vi "TestSpeedCache.vi"() -> ()   [LabVIEW 2017]
uses:
  <vilib>/addons/InsightCM/Utilities/Analysis/Shared/controls/SpeedCache.ctl
  <vilib>/addons/InsightCM/Utilities/Analysis/Shared/controls/SpeedCacheOps.ctl
  <vilib>/addons/InsightCM/Utilities/Analysis/Shared/AnalysisHelper.lvlib
panel:
  out "speed (RPM) 11":dbl
  out "pulse cache 11":T1
  in  "pulse position data 11":dbl[](array[numeric])
  out "speed (RPM) 10":dbl
  out "speed (RPM) 9":dbl
  out "pulse cache 10":T1
  out "pulse cache 9":T1
  in  "pulse position data 10":dbl[](array[numeric])
  in  "pulse position data 9":dbl[](array[numeric])
  out "pulse cache":T1
  out "Speed (RPM) 8":dbl
  out "Pulse Cache Type 8":T1
  in  "pulse position data 8":dbl[](array[numeric])
  in  "pulse position data 7":dbl[](array[numeric])
  out "Speed (RPM) 7":dbl
  out "Pulse Cache Type 7":T1
  out "Pulse Cache Type 6":T1
  out "Pulse Cache Type 5":T1
  out "Pulse Cache Type 4":T1
  out "Pulse Cache Type 3":T1
  out "Pulse Cache Type 2":T1
  out "Pulse Cache Type":T1
  out "Speed (RPM) 6":dbl
  out "Speed (RPM) 5":dbl
  out "Speed (RPM) 4":dbl
  in  "pulse position data 6":dbl[](array[numeric])
  in  "pulse position data 5":dbl[](array[numeric])
  in  "pulse position data 4":dbl[](array[numeric])
  out "Speed (RPM) 3":dbl
  out "Speed (RPM) 2":dbl
  out "Speed (RPM)":dbl
  in  "pulse position data 3":dbl[](array[numeric])
  in  "pulse position data 2":dbl[](array[numeric])
  in  "pulse position data":dbl[](array[numeric])
  # "120"
  # "40"
  # "30"
  # "40"
  # "24"
  # "20"
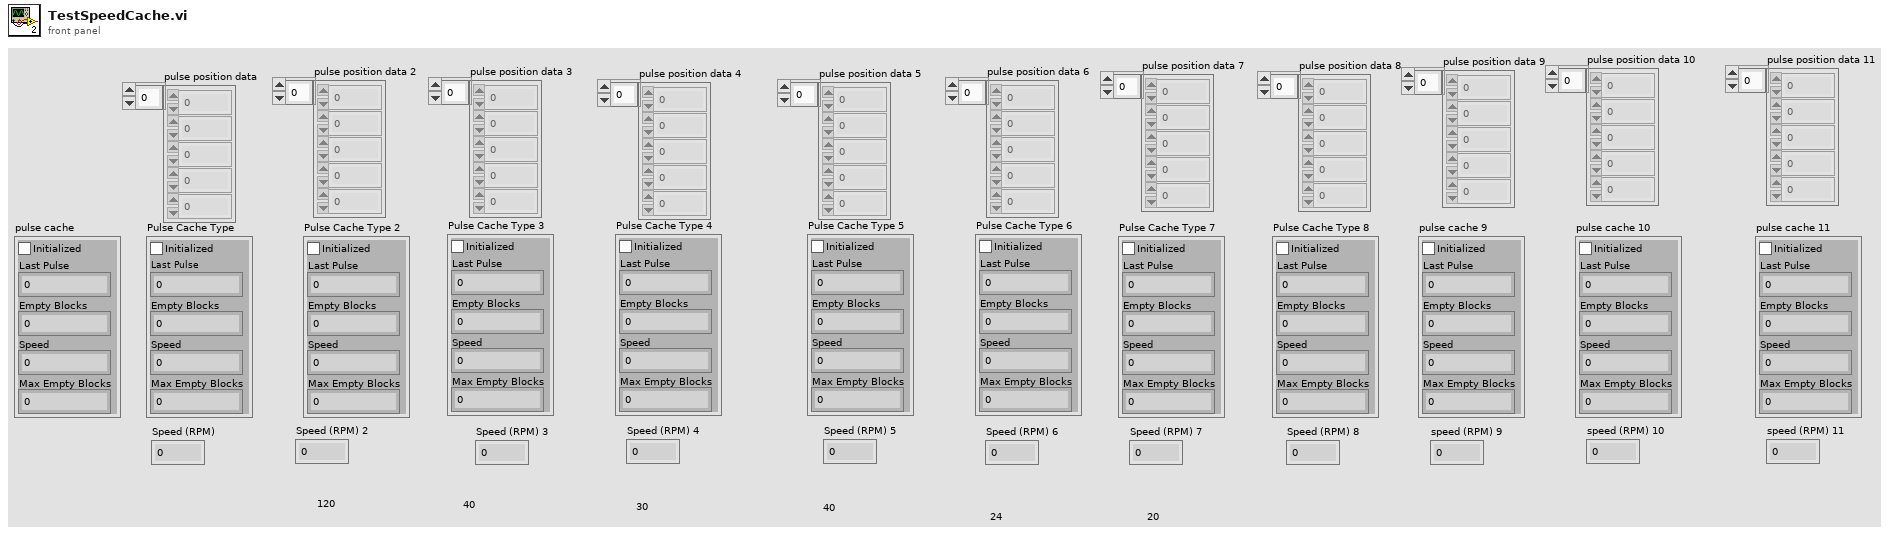
[diagram p1: front panel]
types:
  T1 = typedef "AnalysisHelper.lvlib/SpeedCache.ctl" = cluster{"Initialized":bool, "Last Pulse":dbl, "Empty Blocks":i32, "Speed":dbl, "Max Empty Blocks":i32}
  T2 = typedef "AnalysisHelper.lvlib/SpeedCacheOps.ctl" = enum16{"Init", "GetSpeed"}
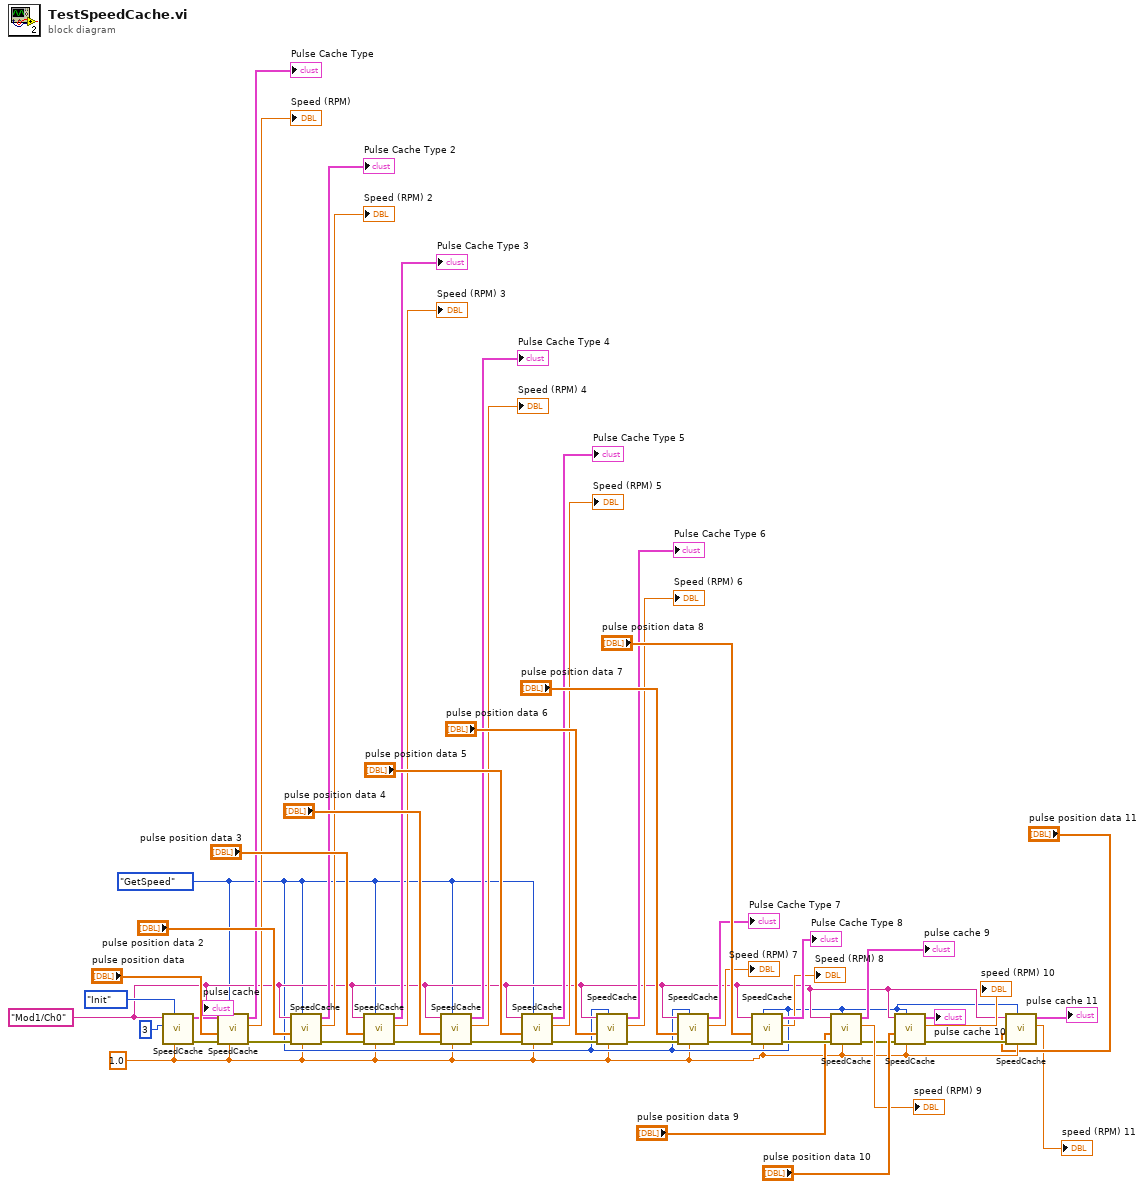
[diagram p0: block diagram]
diagram:
  w6 = SpeedCacheOps."GetSpeed" ("operation")
  w5 = 1.0 ("size of this data block")
  w7 = "Mod1/Ch0" ("channel")
  n1 = call <vilib>:"SpeedCache.vi"("size of this data block"=w5, "operation"=SpeedCacheOps."Init", "max empty blocks"=3, "channel"=w7) -> ("error out"=w49:errorcluster, "pulse cache"=→"pulse cache":T1)  [unwired: 5 in, 1 out]
  n2 = call <vilib>:"SpeedCache.vi"("size of this data block"=w5, "operation"=w6, "error in (no error)"=w49, "pulse position data"="pulse position data", "channel"=w7) -> ("error out"=w23:errorcluster, "speed (RPM)"=→"Speed (RPM)":dbl, "pulse cache"=→"Pulse Cache Type":T1)  [unwired: 4 in]
  n3 = call <vilib>:"SpeedCache.vi"("size of this data block"=w5, "operation"=w6, "error in (no error)"=w23, "pulse position data"="pulse position data 2", "channel"=w7) -> ("error out"=w22:errorcluster, "speed (RPM)"=→"Speed (RPM) 2":dbl, "pulse cache"=→"Pulse Cache Type 2":T1)  [unwired: 4 in]
  n4 = call <vilib>:"SpeedCache.vi"("size of this data block"=w5, "operation"=w6, "error in (no error)"=w22, "pulse position data"="pulse position data 3", "channel"=w7) -> ("error out"=w21:errorcluster, "speed (RPM)"=→"Speed (RPM) 3":dbl, "pulse cache"=→"Pulse Cache Type 3":T1)  [unwired: 4 in]
  n5 = call <vilib>:"SpeedCache.vi"("size of this data block"=w5, "operation"=w6, "error in (no error)"=w21, "pulse position data"="pulse position data 4", "channel"=w7) -> ("error out"=w20:errorcluster, "speed (RPM)"=→"Speed (RPM) 4":dbl, "pulse cache"=→"Pulse Cache Type 4":T1)  [unwired: 4 in]
  n6 = call <vilib>:"SpeedCache.vi"("size of this data block"=w5, "operation"=w6, "error in (no error)"=w20, "pulse position data"="pulse position data 5", "channel"=w7) -> ("error out"=w19:errorcluster, "speed (RPM)"=→"Speed (RPM) 5":dbl, "pulse cache"=→"Pulse Cache Type 5":T1)  [unwired: 4 in]
  n7 = call <vilib>:"SpeedCache.vi"("size of this data block"=w5, "operation"=w6, "error in (no error)"=w19, "pulse position data"="pulse position data 6", "channel"=w7) -> ("error out"=w18:errorcluster, "speed (RPM)"=→"Speed (RPM) 6":dbl, "pulse cache"=→"Pulse Cache Type 6":T1)  [unwired: 4 in]
  n8 = call <vilib>:"SpeedCache.vi"("size of this data block"=w5, "operation"=w6, "error in (no error)"=w18, "pulse position data"="pulse position data 7", "channel"=w7) -> ("error out"=w17:errorcluster, "speed (RPM)"=→"Speed (RPM) 7":dbl, "pulse cache"=→"Pulse Cache Type 7":T1)  [unwired: 4 in]
  n9 = call <vilib>:"SpeedCache.vi"("size of this data block"=w5, "operation"=w6, "error in (no error)"=w17, "pulse position data"="pulse position data 8", "channel"=w7) -> ("error out"=w15:errorcluster, "speed (RPM)"=→"Speed (RPM) 8":dbl, "pulse cache"=→"Pulse Cache Type 8":T1)  [unwired: 4 in]
  n10 = call <vilib>:"SpeedCache.vi"("size of this data block"=w5, "operation"=w6, "error in (no error)"=w15, "pulse position data"="pulse position data 9", "channel"=w7) -> ("error out"=w8:errorcluster, "speed (RPM)"=→"speed (RPM) 9":dbl, "pulse cache"=→"pulse cache 9":T1)  [unwired: 4 in]
  n11 = call <vilib>:"SpeedCache.vi"("size of this data block"=w5, "operation"=w6, "error in (no error)"=w8, "pulse position data"="pulse position data 10", "channel"=w7) -> ("error out"=w4:errorcluster, "speed (RPM)"=→"speed (RPM) 10":dbl, "pulse cache"=→"pulse cache 10":T1)  [unwired: 4 in]
  n12 = call <vilib>:"SpeedCache.vi"("size of this data block"=w5, "operation"=w6, "error in (no error)"=w4, "pulse position data"="pulse position data 11", "channel"=w7) -> ("speed (RPM)"=→"speed (RPM) 11":dbl, "pulse cache"=→"pulse cache 11":T1)  [unwired: 4 in, 1 out]
